vi "Main.vi"() -> ()   [LabVIEW 2020]
doc: "Ce VI modèle est conçu pour le modèle de conception Gestionnaire de messages dans une file d'attente.\n\nLa boucle de gestion d'événements génère des messages en fonction des actions sur l'interface utilisateur.\n\nLa boucle de gestion de messages traite les messages générés par la boucle de gestion d'événements ou par d'autres messages. Les messages sont des valeurs chaîne ; il est donc facile d'ajouter de nouveaux messages à la structure condition Conditions de messages de la boucle de gestion de messages Chaque cluster Message peut en outre fournir une valeur optionnelle pour Données de message, un variant qui peut être converti aux données requises pour un message spécifique."
uses:
  controls/Ctrl_RefPad.ctl
  support/Message Queue/Enqueue Message (Single).vi
  support/Message Queue/Message Queue.lvlib
  support/User Event - Stop/User Event - Stop.lvlib
panel:
  in  "Btn_Error_etat":bool caption="Error state"
  in  "Btn_Error":bool caption="Error"
  out "sortie d'erreur":errorcluster
  out "Display":cluster{"Num":dbl, "Char":string}
  in  "Pad":T1
  in  "Btn_Stop":bool
  # "Calculatrice"
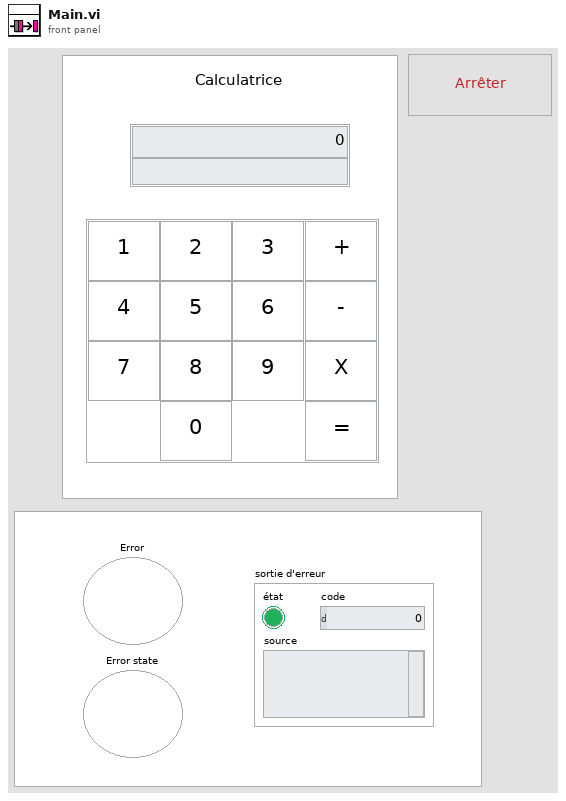
[diagram p1: front panel]
types:
  T1 = cluster{"Btn_1":bool, "Btn_2":bool, "Btn_3":bool, "Btn_4":bool, "Btn_5":bool, "Btn_6":bool, "Btn_7":bool, "Btn_8":bool, "Btn_9":bool, "Btn_0":bool, "Btn_+":bool, "Btn_-":bool, "Btn_X":bool, "Btn_=":bool}
  T2 = cluster{"état":bool, "code":i32, "source":string}
  T3 = typedef "Message Queue.lvlib/All Message Queues.ctl" = cluster{"Conductor":refnum<queue>, "IU":refnum<queue>}
  T4 = typedef "Ctrl_RefPad.ctl" = cluster{"BTN_Ref":refnum<vi>, "CharPad":string}
  T5 = typedef "UI Data.ctl" = cluster{"Fifo":T3, "UI":T6, "Event":cluster{"Stop":refnum<user-event>}, "Data":cluster{"Display":cluster{"Num":dbl, "Char":string}, "memory":string}}
  T6 = typedef "ctrl_UI_Ref.ctl" = cluster{"Display":refnum<vi>}
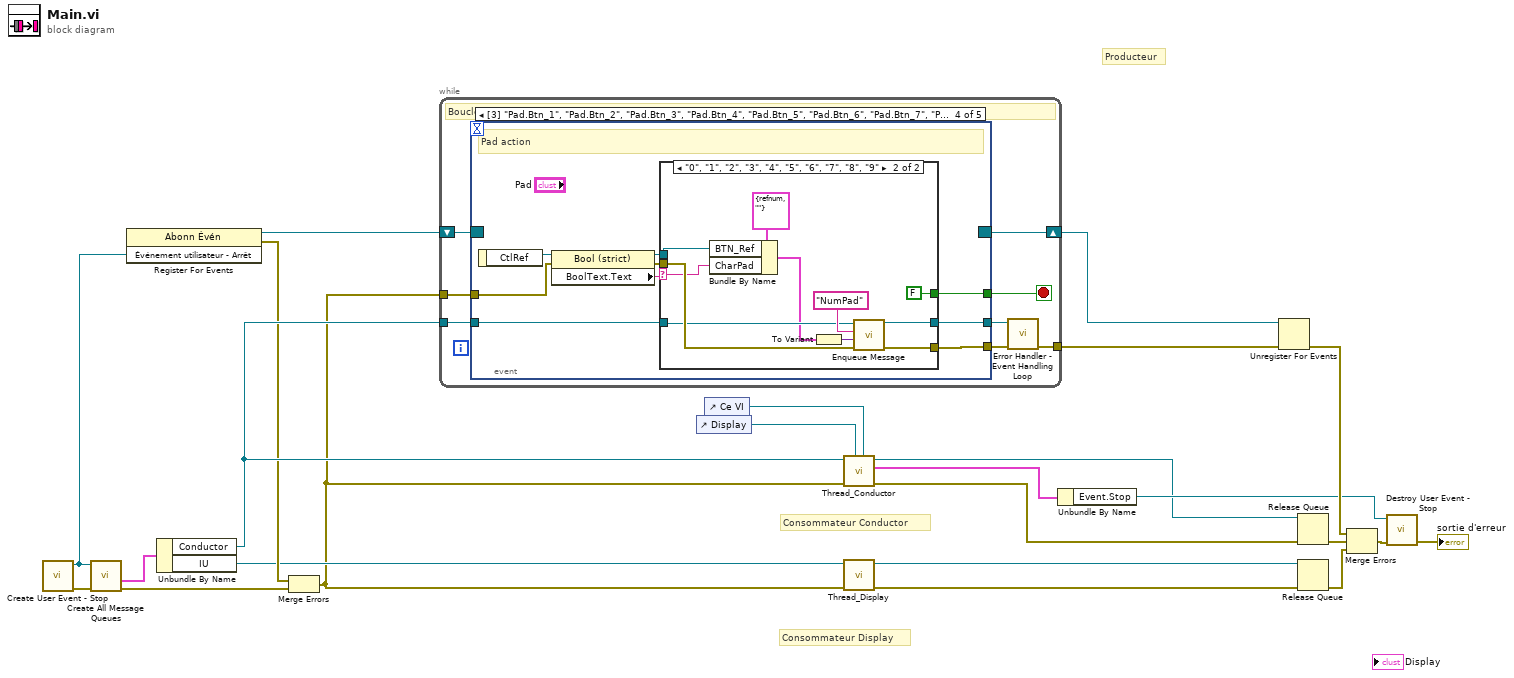
[diagram p0: block diagram]
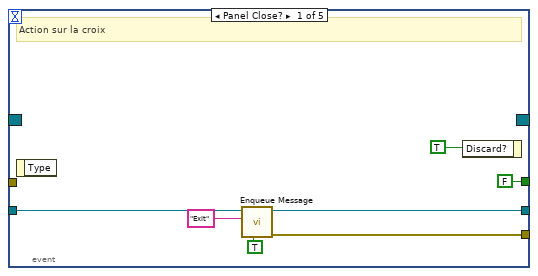
[diagram p2: hidden frame]
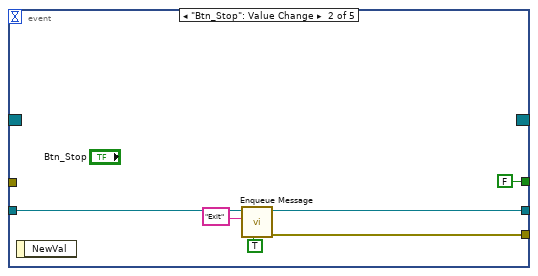
[diagram p3: hidden frame]
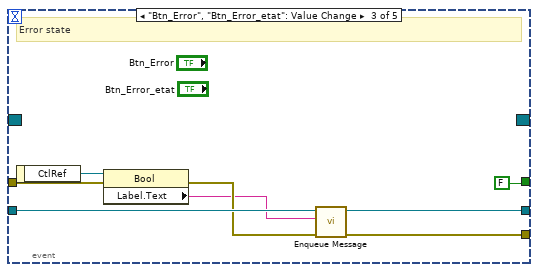
[diagram p4: hidden frame]
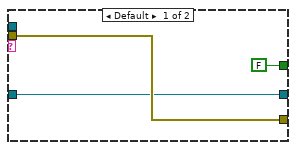
[diagram p5: hidden frame]
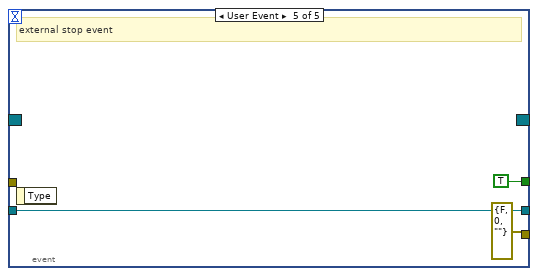
[diagram p6: hidden frame]
diagram:
  # "Producteur"
  # "Consommateur Display"
  # "Consommateur Conductor"
  n1 = call "Create User Event - Stop.vi"() -> ("error out"=w21:T2, "Événement utilisateur - Arrêt"=w14:refnum<user-event>)  [unwired: 10 in]
  n2 = call "Create All Message Queues.vi"("error in (no error)"=w21, "Stop Event"=w14) -> ("error out"=w24:T2, "Fifo"=w23:T3)  [unwired: 8 in]
  n3 = register-events(w14) -> (reference out=w16:refnum<event-registration>, error out=w15:errorcluster)  [unwired: 2 in]
  n4 = Unbundle By Name(w23) -> ("Conductor"=w22:refnum<queue>, "IU"=w8:refnum<queue>)
  n5 = Merge Errors(w15, w24) -> (w7:errorcluster)
  n6 = while {
    tunnel: w22 -> [w32]
    shift-right: [w30] -> w18
    shift-left: w16 -> [w31]
    tunnel: [w26] -> w17
    tunnel: w7 -> [w25]
    stop <- w28 stop-if-true
    # "Boucle de gestion d'événements"
    n7 = event shown="[3] \"Pad.Btn_1\", \"Pad.Btn_2\", \"Pad.Btn_3\", \"Pad.Btn_4\", \"Pad.Btn_5\", \"Pad.Btn_6\", \"Pad.Btn_7\", \"Pad.Btn_8\", \"Pad.Btn_9\", \"Pad.Btn_0\", \"Pad.Btn_+\": Valeur changée" {
      selector: w31 -> [_ _ _ _ _]
      dyn-events: [_ _ _ _ _] -> w30
      timeout: _ -> [_ _ _ _ _]
      tunnel: [FALSE ("Discard?") FALSE ("Discard?") FALSE w55 TRUE ("Discard?")] -> w28
      tunnel: w32 -> [w38 w45 w51 w57 w79]
      tunnel: [w37 w44 w46 w58 T2 {"état"=FALSE, "code"=0, "source"=""} ("error out")] -> w29
      tunnel: [w36 w43 w50 w56 w79] -> w27
      tunnel: w25 -> [_ _ w52 w61 _]
      event Panel Close? {
        # "Action sur la croix"
        n8 = event-data() -> ()  [unwired: 1 in, 1 out]
        n9 = call-poly "Enqueue Message.vi"("Message prioritaire ? (F)"=TRUE ("Priority Message? (F)"), "Message"="Exit", "File d'attente de messages"=w38) -> ("error out"=w37:T2, "File d'attente de message dup."=w36:refnum<queue>)  [unwired: 7 in]
        n10 = event-data ("Event Filter Node")("Discard?"=TRUE) -> ()  [unwired: 1 in, 1 out]
      }
      event "Btn_Stop": Value Change {
        n11 = event-data() -> ()  [unwired: 1 in, 1 out]
        n12 = call-poly "Enqueue Message.vi"("Message prioritaire ? (F)"=TRUE ("Priority Message? (F)"), "Message"="Exit", "File d'attente de messages"=w45) -> ("error out"=w44:T2, "File d'attente de message dup."=w43:refnum<queue>)  [unwired: 7 in]
      }
      event "Btn_Error", "Btn_Error_etat": Value Change {
        # "Error state"
        n13 = event-data() -> ("CtlRef"=w53:refnum<vi>)  [unwired: 1 in]
        n14 = property class="Bool"(reference=w53, error in=w52) -> (error out=w49:errorcluster, "Label.Text"=w48:string)  [unwired: 1 out]
        n15 = call-poly "Enqueue Message.vi"("error in (no error)"=w49, "Message"=w48, "File d'attente de messages"=w51) -> ("error out"=w46:T2, "File d'attente de message dup."=w50:refnum<queue>)  [unwired: 7 in]
      }
      event "Pad.Btn_1", "Pad.Btn_2", "Pad.Btn_3", "Pad.Btn_4", "Pad.Btn_5", "Pad.Btn_6", "Pad.Btn_7", "Pad.Btn_8", "Pad.Btn_9", "Pad.Btn_0", "Pad.Btn_+": Value Change {
        # "Pad action"
        n16 = event-data() -> ("CtlRef"=w62:refnum<vi>)  [unwired: 1 in]
        n17 = property class="Bool (strict)"(reference=w62, error in=w61) -> (reference out=w54:refnum<vi>, error out=w59:errorcluster, "BoolText.Text"=w60:string)
        n18 = case shown="\"0\", \"1\", \"2\", \"3\", \"4\", \"5\", \"6\", \"7\", \"8\", \"9\"" w60 {
          selector: w60 -> [_ w68]
          tunnel: w59 -> [w65 w75]
          tunnel: [w65 w74] -> w58
          tunnel: w57 -> [w64 w72]
          tunnel: [w64 w71] -> w56
          tunnel: [FALSE FALSE] -> w55
          tunnel: w54 -> [_ w69]
          frame Default {
          }
          frame "0", "1", "2", "3", "4", "5", "6", "7", "8", "9" {
            n19 = Bundle By Name(cluster=T4 {"BTN_Ref"=refnum, "CharPad"=""}, "BTN_Ref"=w69, "CharPad"=w68) -> (w67:T4)
            n20 = To Variant(anything=w67) -> (Variant=w73:variant)
            n21 = call-poly "Enqueue Message.vi"("error in (no error)"=w75, "Données de message"=w73, "Message"="NumPad", "File d'attente de messages"=w72) -> ("error out"=w74:T2, "File d'attente de message dup."=w71:refnum<queue>)  [unwired: 6 in]
          }
        }
      }
      event User Event {
        # "external stop event"
        n22 = event-data() -> ()  [unwired: 1 in, 1 out]
      }
    }
    n23 = call "Error Handler - Event Handling Loop.vi"("error in (no error)"=w29, "File d'attente de messages"=w27) -> ("erreur en entrée dup."=w26:T2)  [unwired: 8 in, 1 out]
  }
  n24 = control-ref of="Display"() -> (w1:refnum<vi>)
  n25 = control-ref of="Ce VI"() -> (w2:refnum<vi>)
  n26 = call "Thread_Conductor.vi"("Ce VI"=w2, "Display"=w1, "entrée d'erreur (pas d'erreur)"=w7, "File d'attente en entrée"=w22) -> ("error out"=w10:errorcluster, "Data Cluster"=w13:T5, "File d'attente en sortie"=w11:refnum<queue>)  [unwired: 5 in]
  n27 = call "Thread_Display.vi"("entrée d'erreur (pas d'erreur)"=w7, "File d'attente en entrée"=w8) -> ("sortie d'erreur"=w6:errorcluster, "File d'attente en sortie"=w5:refnum<queue>)  [unwired: 8 in]
  n28 = Unbundle By Name(w13) -> ("Event.Stop"=w12:refnum<user-event>)
  n29 = Unregister For Events(event registration refnum=w18, error in=w17) -> (error out=w19:errorcluster)
  n30 = Release Queue(queue=w11, error in (no error)=w10) -> (error out=w9:errorcluster)  [unwired: 1 in, 2 out]
  n31 = Release Queue(queue=w5, error in (no error)=w6) -> (error out=w4:errorcluster)  [unwired: 1 in, 2 out]
  n32 = Merge Errors(w19, w9, w4) -> (w20:errorcluster)
  n33 = call "Destroy User Event - Stop.vi"("error in (no error)"=w20, "Événement utilisateur - Arrêt"=w12) -> ("error out"=→"sortie d'erreur":T2)  [unwired: 9 in]
